vi "Initialize OAuth for Facebook.vi"(9 "Scopes":string[](array[string])=["public_profile"], 10 "Client Secret":string, 11 "Client ID":string) -> (3 "Oauth2.Facebook":refnum<class "Oauth2.Facebook.lvclass">)   [LabVIEW 2013, in "Oauth2.Facebook.lvclass"]
uses:
  Oauth2.Facebook.lvclass
  Oauth2/Oauth2.lvclass
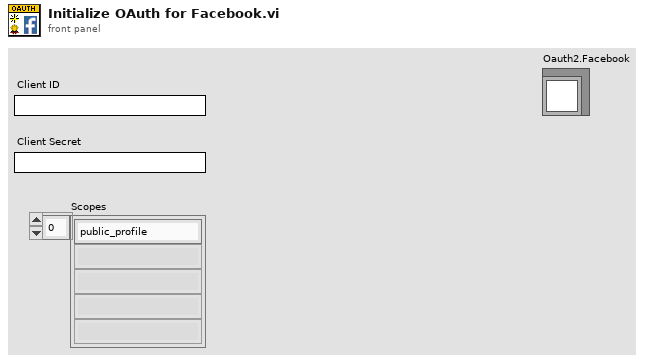
[diagram p1: front panel]
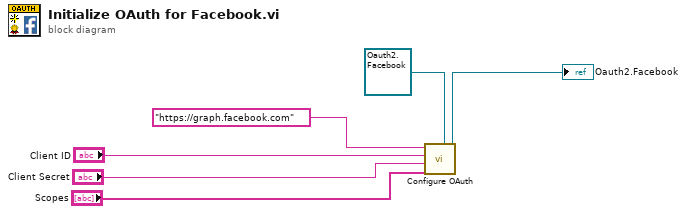
[diagram p0: block diagram]
diagram:
  n1 = call "Configure OAuth.vi"("Oauth2 in"=refnum<class "Oauth2.Facebook.lvclass"> refnum ("Oauth2.GitHub in"), "scopes"="Scopes", "Client Secret"="Client Secret", "Client ID"="Client ID", "Authorization Server URI"="https://graph.facebook.com") -> ("Oauth2"=→"Oauth2.Facebook":refnum<class "Oauth2.Facebook.lvclass">)  [unwired: 5 in, 1 out]
